vi "Untitled 6 (SubVI).vi"(10 "Кол-во копий":i32, 11 "Array":dbl[](array[numeric])) -> (2 "см. 1.5":dbl[][](array[numeric]), 3 "Numeric":i32)   [LabVIEW 2017]
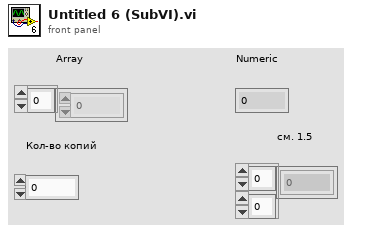
[diagram p1: front panel]
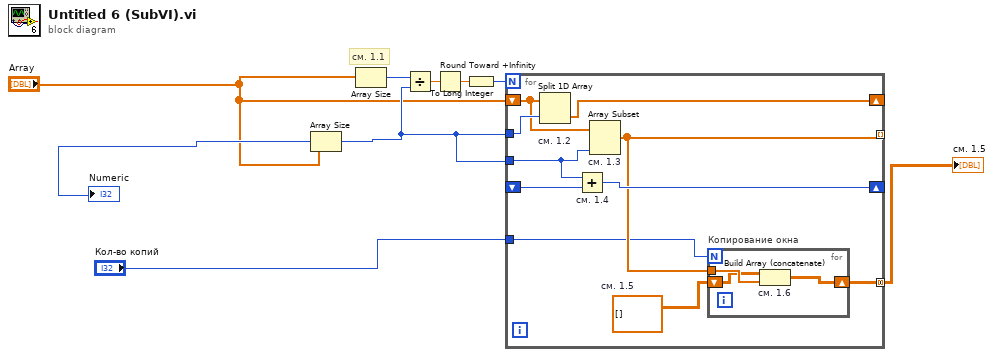
[diagram p0: block diagram]
diagram:
  # "см. 1.1"
  n1 = Array Size(array="Array") -> (size(s)=w7:i32)
  "Numeric" <- w7
  n2 = Array Size(array="Array") -> (size(s)=w1:i32)
  n3 = Divide(x=w1, y=w7) -> (x/y=w2:dbl)
  n4 = Round Toward +Infinity(x=w2) -> (ceil(x): smallest int >= x=w3:dbl)
  n5 = To Long Integer(number=w3) -> (32bit integer=w4:i32)
  n6 = for {
    N: w4 -> [_]
    shift-right: [w18] -> _
    shift-left: "Array" -> [w16]
    tunnel: w7 -> [w17]
    shift-right: [w14] -> _
    shift-left: _ -> [w13]
    tunnel: w7 -> [w15]
    tunnel: [w12] -> _ mode=indexing
    tunnel: [w11] -> w8 mode=concatenating
    tunnel: "Кол-во копий" -> [w9]
    w10 = dbl[][] []  # см. 1.5
    n7 = Split 1D Array "см. 1.2"(array=w16, index=w17) -> (second subarray=w18:dbl[])  [unwired: 1 out]
    n8 = Add "см. 1.4"(x=w15, y=w13) -> (x+y=w14:i32)
    n9 = Array Subset "см. 1.3"(array=w16, length=w15) -> (w12:dbl[])  [unwired: 1 in]
    n10 = for "Копирование окна" {
      N: w9 -> [_]
      tunnel: w12 -> [w20]
      shift-right: [w21] -> w11
      shift-left: w10 -> [w19]
      n11 = Build Array (concatenate) "см. 1.6"(w19, w20) -> (w21:dbl[][])
    }
  }
  "см. 1.5" <- w8
